vi "Motor-Open.vi"(0 "S/N Motor":string(combo)) -> (1 "MG17Motor 2":refnum<k7>, 2 "error out":errorcluster)   [LabVIEW 2014]
doc: "André Romero - 2019\nandretec@ifsc.usp.br\nIFSC - USP"
panel:
  in  "MG17Motor":refnum<k7>(container)
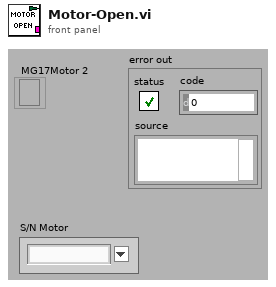
[diagram p1: front panel]
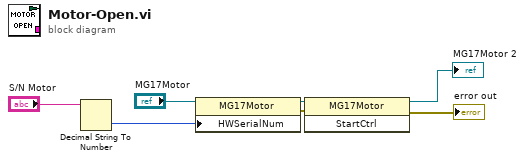
[diagram p0: block diagram]
diagram:
  n1 = Decimal String To Number(string="S/N Motor") -> (number=w2:i32)  [unwired: 2 in, 1 out]
  n2 = property class="MG17Motor"(reference="MG17Motor", "HWSerialNum"=w2) -> (reference out=w3:refnum<k7>, error out=w4:errorcluster)  [unwired: 1 in]
  n3 = invoke class="MG17Motor" method="StartCtrl"(reference=w3, error in=w4) -> (reference out=→"MG17Motor 2":refnum<k7>, error out=→"error out":errorcluster)  [unwired: 1 in, 1 out]
